vi "RW_test.vi"(11 "VISAsession":refnum<visa-resource-name>="wavefactoryU10") -> (0 "error out":errorcluster caption="Error OUT")   [LabVIEW 2018]
panel:
  in  "write buffer 2":string=":chan1:freq?; :chan2:freq?; :chan1:volt?; :chan2:volt?; :chan1:phase?; :chan2:phase?"
  in  "read":bool=TRUE
  in  "write buffer":string="chan1:volt?;:chan2:volt?"
  out "read buffer":string="02.000E+00;02.000E+00\r\n"
  out "elapsed time (ms)":u32=48
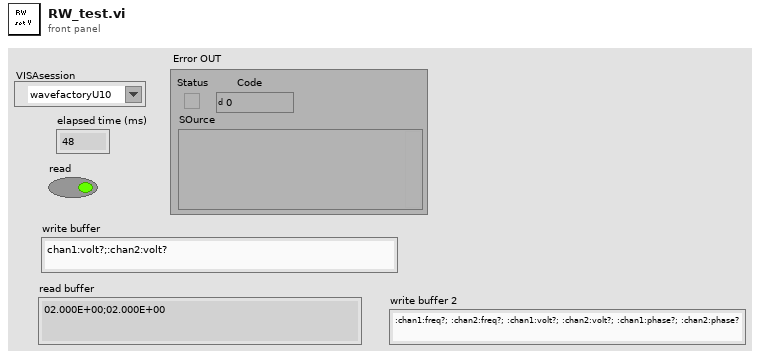
[diagram p1: front panel]
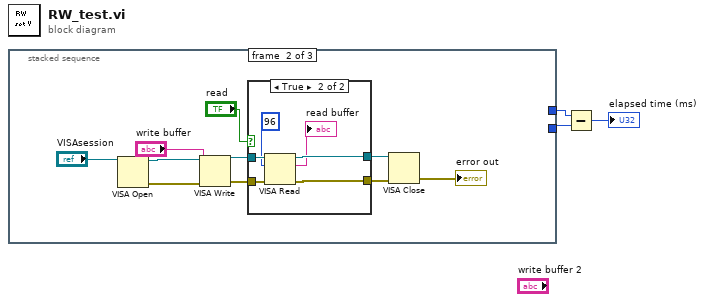
[diagram p0: block diagram]
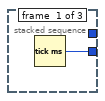
[diagram p2: hidden frame]
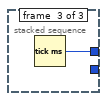
[diagram p4: hidden frame]
diagram:
  n1 = stacked-sequence {
    tunnel: [w4 _ _] -> w2
    tunnel: [_ _ w23] -> w3
    frame #0 {
      n2 = Tick Count (ms)() -> (millisecond timer value=w4:u32)
    }
    frame #1 {
      n3 = VISA Open(VISA resource name="VISAsession") -> (VISA resource name=w13:refnum<visa-resource-name>, error out=w14:errorcluster)  [unwired: 4 in]
      n4 = VISA Write(VISA resource name=w13, write buffer="write buffer", error in (no error)=w14) -> (VISA resource name out=w10:refnum<visa-resource-name>, error out=w9:errorcluster)  [unwired: 1 out]
      n5 = case shown="True" "read" {
        tunnel: w10 -> [w16 w22]
        tunnel: w9 -> [w15 w21]
        tunnel: [w16 w20] -> w8
        tunnel: [w15 w19] -> w7
        frame False {
        }
        frame True {
          n6 = VISA Read(VISA resource name=w22, byte count=u32 96, error in (no error)=w21) -> (VISA resource name out=w20:refnum<visa-resource-name>, read buffer=→"read buffer":string, error out=w19:errorcluster)  [unwired: 1 out]
        }
      }
      n7 = VISA Close(VISA resource name=w8, error in (no error)=w7) -> (error out=→"error out":errorcluster)
    }
    frame #2 {
      n8 = Tick Count (ms)() -> (millisecond timer value=w23:u32)
    }
  }
  n9 = Subtract(x=w3, y=w2) -> (x-y=→"elapsed time (ms)":u32)
